vi "Init Data.vi"(10 "Data":T1) -> (3 "Msg out":refnum<class "Msg.lvclass">)   [LabVIEW 2020, in "TcpClientList.lvlib" / "Msg.lvclass"]
uses:
  Msg.lvclass
  Data.ctl
  TcpClientInfo/Data.ctl
  Msg.lvclass/Msg.ctl
  TcpClientList.lvlib
  TcpClientInfo/TcpClientInfo.lvlib
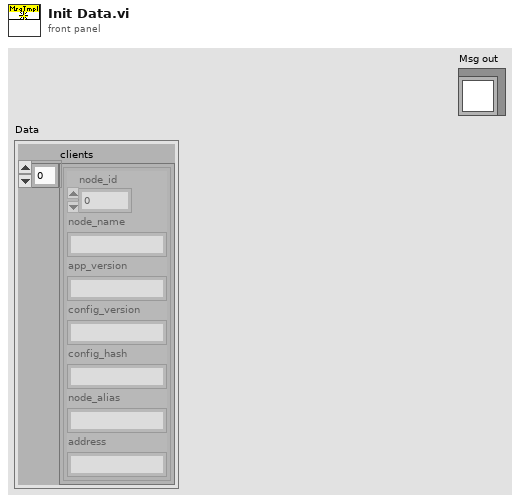
[diagram p1: front panel]
types:
  T1 = typedef "TcpClientList.lvlib/Data.ctl" = cluster{"clients":T2[]}
  T2 = typedef "TcpClientInfo.lvlib/Data.ctl" = cluster{"node_id":u32, "node_name":string, "app_version":string, "config_version":string, "config_hash":string, "node_alias":string, "address":string}
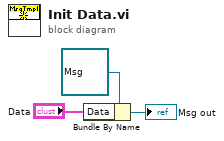
[diagram p0: block diagram]
diagram:
  n1 = Bundle By Name(cluster=refnum<class "Msg.lvclass"> refnum ("Msg out"), "Data"="Data") -> (→"Msg out":refnum<class "Msg.lvclass">)
